vi "PC_Main.vi"() -> ()   [LabVIEW 2017]
uses:
  <vilib>/userdefined/High Color/IMAQdx.ctl
  <vilib>/vision/driver/NI_Vision_Acquisition_Software.lvlib
  <vilib>/vision/NI_Vision_Development_Module.lvlib
panel:
  out "Object Centre Array":cluster{"X":dbl, "Y":dbl}[](array[cluster])
  out "Particle Reports (Pixels)":T1(array[cluster]) {"Orientation" format="%.2f"; "Dimensions"."Height" format="%.2f"; "Dimensions"."Width" format="%.2f"; "Center of Mass"."Y" format="%.2f"; "Center of Mass"."X" format="%.2f"; "Bounding Rect"."Bottom" format="%.2f"; "Bounding Rect"."Right" format="%.2f"; "Bounding Rect"."Top" format="%.2f"; "Bounding Rect"."Left" format="%.2f"; "Number of Holes" format="%.2f"; "Area" format="%.2f"}
  in  "Method (clustering)":i32(ring) items=["clustering", "entropy", "metric", "moments", "inter-class variance"]
  in  "File Path":path=path "\\\\hs6.lboro.ac.uk\\eltpwq/GitHub/mechatronics/LabVIEW/calibration6.png"
  in  "Number of Erosion":i32=6
  in  "Color Plane":i32(ring)=1 items=["Red", "Green", "Blue", "Hue", "Saturation", "Luminance", "Value", "Intensity"]
  in  "Angle (degrees)":sgl format="%.2f"
  in  "Mirror":bool=TRUE
  in  "Symmetry":u32(ring)=1 items=["Horizontal", "Vertical", "Central", "1st Diagonal", "2nd Diagonal"]
  in  "Camera":T2="cam1"
  out "Image":T3(plugin-control)
  in  "stop":bool
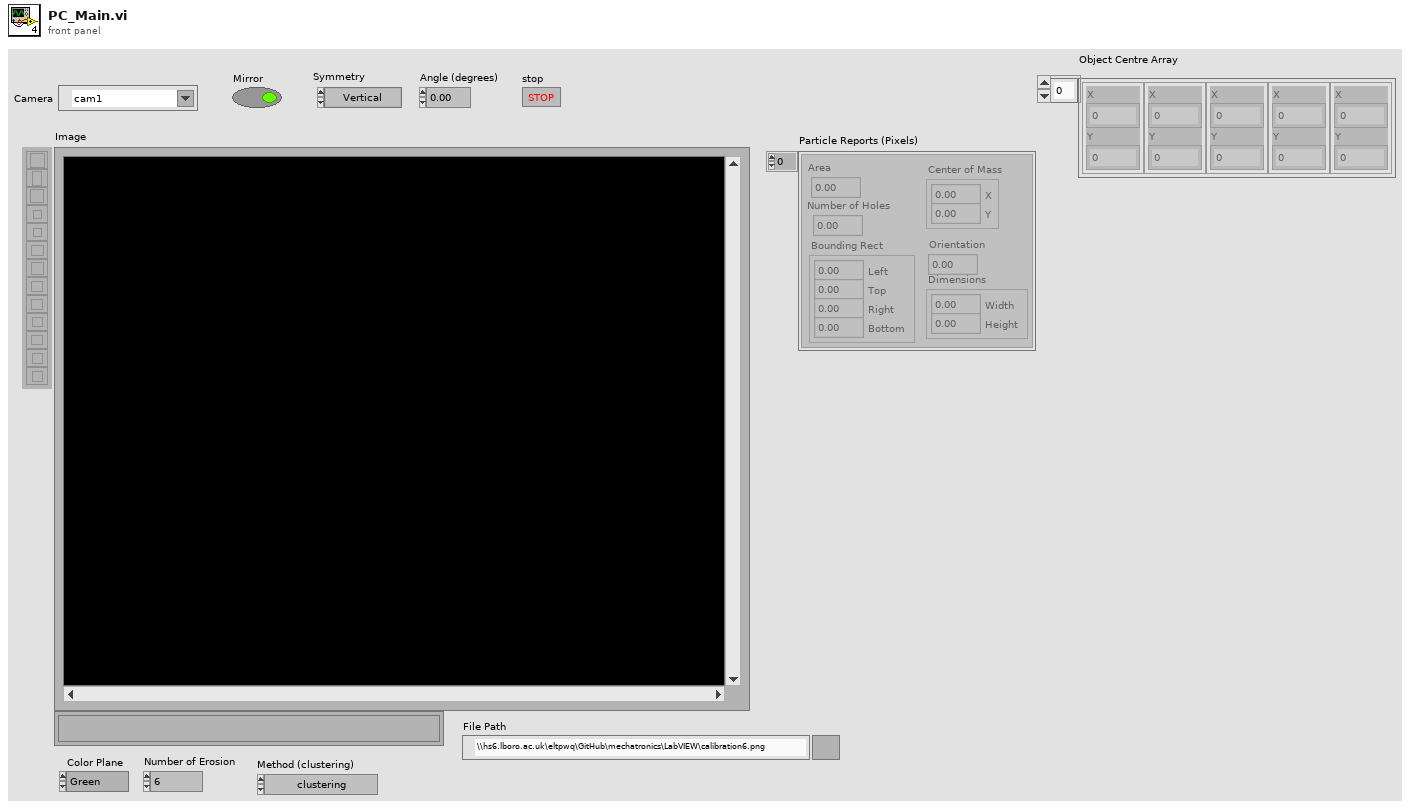
[diagram p1: front panel]
types:
  T1 = cluster{"Area":dbl, "Number of Holes":dbl, "Bounding Rect":cluster{"Left":dbl, "Top":dbl, "Right":dbl, "Bottom":dbl}, "Center of Mass":cluster{"X":dbl, "Y":dbl}, "Orientation":dbl, "Dimensions":cluster{"Width":dbl, "Height":dbl}}[]
  T2 = typedef "IMAQdx.ctl" = refnum<k21>
  T3 = typedef "IMAQ Image.ctl" = refnum<image>
  T4 = typedef "Image Type" = u32
  T5 = enum8{"Enabled", "Disabled", "Disabled and Grayed Out"}
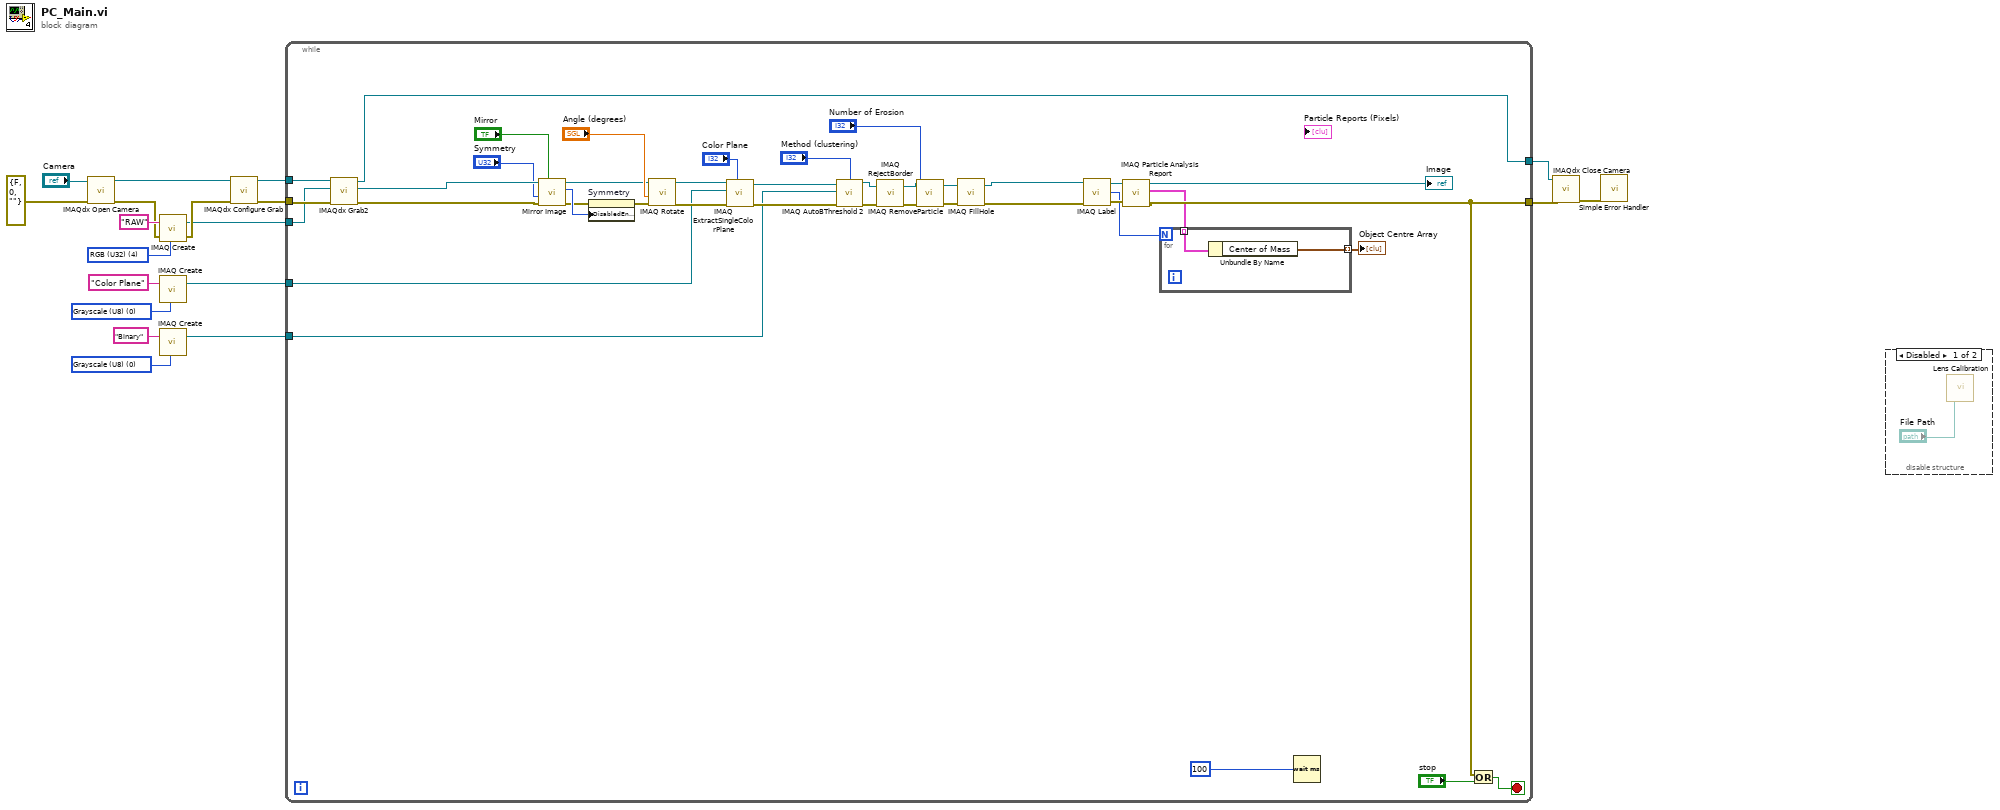
[diagram p0: block diagram]
diagram:
  w3 = T4 0 items=["Grayscale (U8)", "Grayscale (I16)", "Grayscale (SGL)", "Complex (CSG)", "RGB (U32)", "HSL (U32)", "RGB (U64)", "Grayscale (U16)"] ("Image Type")
  w4 = T4 0 items=["Grayscale (U8)", "Grayscale (I16)", "Grayscale (SGL)", "Complex (CSG)", "RGB (U32)", "HSL (U32)", "RGB (U64)", "Grayscale (U16)"] ("Image Type")
  w17 = T4 4 items=["Grayscale (U8)", "Grayscale (I16)", "Grayscale (SGL)", "Complex (CSG)", "RGB (U32)", "HSL (U32)", "RGB (U64)", "Grayscale (U16)"] ("Image Type")
  n1 = call <vilib>:"IMAQdx Open Camera.vi"("error in"=errorcluster {"status"=FALSE, "code"=0, "source"=""}, "Session In"="Camera") -> ("error out"=w5:errorcluster, "Session Out"=w15:T2)  [unwired: 8 in]
  n2 = call "IMAQ Create"("Image Name"="RAW", "Image Type"=w17, "error in (no error)"=w5) -> ("New Image"=w12:T3, "error out"=w18:errorcluster)  [unwired: 2 in]
  n3 = call "IMAQ Create"("Image Name"="Color Plane", "Image Type"=w4) -> ("New Image"=w6:T3)  [unwired: 3 in, 1 out]
  n4 = call "IMAQ Create"("Image Name"="Binary", "Image Type"=w3) -> ("New Image"=w1:T3)  [unwired: 3 in, 1 out]
  n5 = call <vilib>:"IMAQdx Configure Grab.vi"("error in"=w18, "Session In"=w15) -> ("error out"=w13:errorcluster, "Session Out"=w14:T2)  [unwired: 8 in]
  n6 = while {
    tunnel: w14 -> [w59]
    tunnel: w13 -> [w58]
    tunnel: w12 -> [w57]
    tunnel: [w56] -> w9
    tunnel: [w30] -> w8
    tunnel: w6 -> [w43]
    tunnel: w1 -> [w25]
    stop <- w54 stop-if-true
    n7 = call <vilib>:"IMAQdx Grab2.vi"("error in"=w58, "Image In"=w57, "Session In"=w59) -> ("error out"=w41:errorcluster, "Image Out"=w47:T3, "Session Out"=w56:T2)  [unwired: 5 in, 1 out]
    n8 = call "Mirror Image.vi"("Mirror"="Mirror", "error in (no error)"=w41, "Symmetry"="Symmetry", "Refnum in"=w47) -> ("error out"=w51:errorcluster, "Disabled"=w53:T5, "Refnum out"=w48:T3)  [unwired: 5 in]
    n9 = property on="Symmetry" class="Ring (strict)"(error in=w51, "DisabledEnum"=w53) -> (error out=w52:errorcluster)  [unwired: 1 in, 1 out]
    n10 = call "IMAQ Rotate"("error in (no error)"=w52, "Angle (degrees)"="Angle (degrees)", "Image Src"=w48) -> ("error out"=w44:errorcluster, "Image Dst Out"=w40:T3)  [unwired: 7 in]
    n11 = call "IMAQ ExtractSingleColorPlane"("Color Plane"="Color Plane", "error in (no error)"=w44, "Image Dst"=w43, "Image Src"=w40) -> ("error out"=w38:errorcluster, "Image Dst Out"=w39:T3)  [unwired: 6 in]
    n12 = call "IMAQ AutoBThreshold 2"("Image Src"=w39, "Method (clustering)"="Method (clustering)", "Image Dst"=w25, "error in (no error)"=w38) -> ("Image Dst Out"=w35:T3, "error out"=w37:errorcluster)  [unwired: 9 in, 1 out]
    n13 = call "IMAQ RejectBorder"("error in (no error)"=w37, "Image Src"=w35) -> ("error out"=w33:errorcluster, "Image Dst Out"=w32:T3)  [unwired: 4 in]
    n14 = call "IMAQ RemoveParticle"("error in (no error)"=w33, "Number of Erosion"="Number of Erosion", "Image Src"=w32) -> ("error out"=w28:errorcluster, "Image Dst Out"=w29:T3)  [unwired: 7 in]
    n15 = call "IMAQ FillHole"("error in (no error)"=w28, "Image Src"=w29) -> ("error out"=w21:errorcluster, "Image Dst Out"=w20:T3)  [unwired: 4 in]
    n16 = call "IMAQ Label"("error in (no error)"=w21, "Image Src"=w20) -> ("error out"=w27:errorcluster, "Number of Particles"=w23:i32, "Image Dst Out"=w26:T3)  [unwired: 2 in]
    n17 = call "IMAQ Particle Analysis Report"("error in (no error)"=w27, "Image"=w26) -> ("error out"=w30:errorcluster, "Particle Reports (Pixels)"=w24:T1, "Image Out (duplicate)"=→"Image":T3)  [unwired: 4 in, 3 out]
    n18 = for {
      N: w23 -> [_]
      tunnel: [w61] -> w22 mode=indexing
      tunnel: w24 -> [w60] mode=indexing
      n19 = Unbundle By Name(w60) -> ("Center of Mass"=w61:cluster{"X":dbl, "Y":dbl})
    }
    "Object Centre Array" <- w22
    n20 = Wait (ms)(milliseconds to wait=u32 100) -> ()  [unwired: 1 out]
    n21 = Or(x=w30, y="stop") -> (x .or. y?=w54:bool)
  }
  n22 = call <vilib>:"IMAQdx Close Camera.vi"("error in"=w8, "Session In"=w9) -> ("error out"=w10:errorcluster)  [unwired: 9 in]
  n23 = call <vilib>:"Simple Error Handler.vi"("error in (no error)"=w10) -> ()  [unwired: 4 in, 5 out]
  n24 = disable-structure shown="Disabled" {
    frame Disabled {
      n25 = call "Lens Calibration.vi"("File Path"="File Path") -> ()  [unwired: 5 in, 2 out]
    }
    frame Enabled {
    }
  }
